vi "Write IMAQ Session.vi"(8 "error in (no error)":errorcluster, 9 "IMAQ Session":T1, 10 "Camera Name":string, 11 "Gantry Class in":refnum<class "Gantry.lvclass">) -> (0 "error out":errorcluster, 3 "Gantry Class out":refnum<class "Gantry.lvclass">)   [LabVIEW 2017, in "Gantry.lvclass"]
uses:
  Gantry.lvclass
  <vilib>/userdefined/High Color/IMAQdx.ctl
  Gantry.lvclass/Gantry.ctl
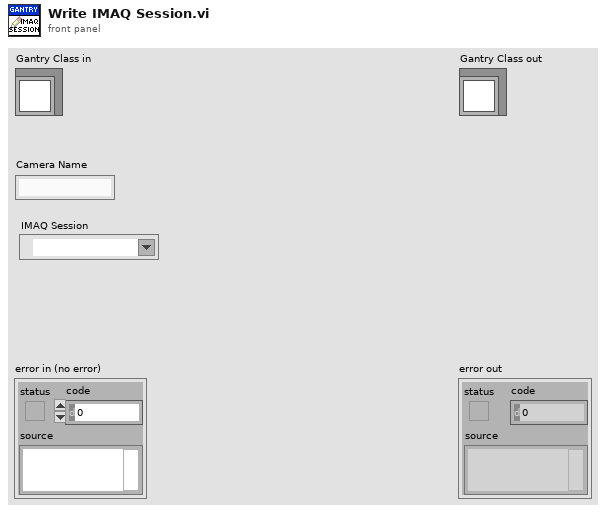
[diagram p1: front panel]
types:
  T1 = typedef "IMAQdx.ctl" = refnum<k21>
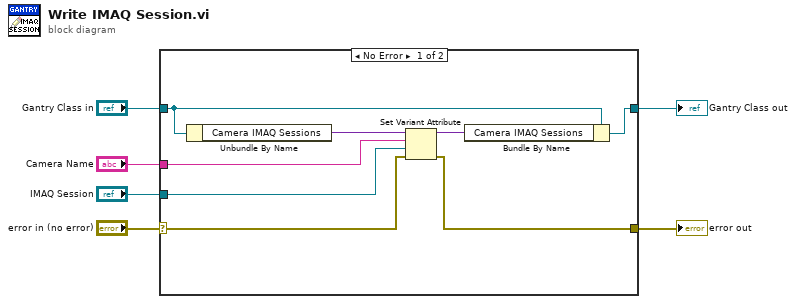
[diagram p0: block diagram]
diagram:
  n1 = case shown="No Error" "error in (no error)" {
    selector: "error in (no error)" -> [w11 w16]
    tunnel: [w10 w16] -> w5
    tunnel: [w8 w15] -> w3
    tunnel: "Gantry Class in" -> [w9 w15]
    tunnel: "Camera Name" -> [w13 _]
    tunnel: "IMAQ Session" -> [w12 _]
    frame No Error {
      n2 = Unbundle By Name(w9) -> ("Camera IMAQ Sessions"=w14:variant)
      n3 = Set Variant Attribute(Variant=w14, name=w13, value=w12, error in=w11) -> (Variant out=w7:variant, error out=w10:errorcluster)  [unwired: 1 out]
      n4 = Bundle By Name(cluster=w9, "Camera IMAQ Sessions"=w7) -> (w8:refnum<class "Gantry.lvclass">)
    }
    frame Error {
    }
  }
  "error out" <- w5
  "Gantry Class out" <- w3
